vi "Configure Measurement.vi"(0 "VISA resource name":refnum<visa-resource-name>, 1 "Manual Resolution (2: 6.5 digits)":enum16{"4.5", "5.5", "6.5", "7.5", "8.5"}(ring)=enum."6.5", 5 "Function (0: DC Voltage)":u16(ring) items=["DC Voltage", "AC Voltage", "AC + DC Voltage", "DC Current", "AC Current", "AC + DC Current", "2-Wire Resistance", "4-Wire Resistance", "Frequency", "Period", "Direct Sampling DC", "Direct Sampling AC", "Sub-Sampling DC", "Sub-Sampling AC"], 7 "Frequency Source (3: AC Voltage)":u16(ring)=3 items=["AC + DC Current", "AC + DC Voltage", "AC Current", "AC Voltage"], 9 "Auto Range (1:ON)":u16(ring)=1 items=["OFF", "ON", "ONCE"], 11 "error in (no error)":errorcluster, 12 "Manual Range (1.00)":dbl=1.0 format="%_3g") -> (4 "VISA resource name out":refnum<visa-resource-name>, 15 "error out":errorcluster)   [LabVIEW 2020, in "3458A Basic Driver.lvlib"]
doc: "Configures the measurement type, resolution, range on the instrument and frequency source. Note that when setting for sub-sampling, you must specify a range, auto range cannot be used with sub-sampling. Also note that setting the integration cycle to a value greater than or equal to one prior to setting the manual resolution will result in the instrument setting the manual resolution to the highest number of digits for the function chosen regardless of user input. So if the user sets the number of integration cycles to one for DCV, the instrument will set the manual resolution to 8.5 digits even if the user sets it to 6.5 digits."
uses:
  3458A Basic Driver.lvlib
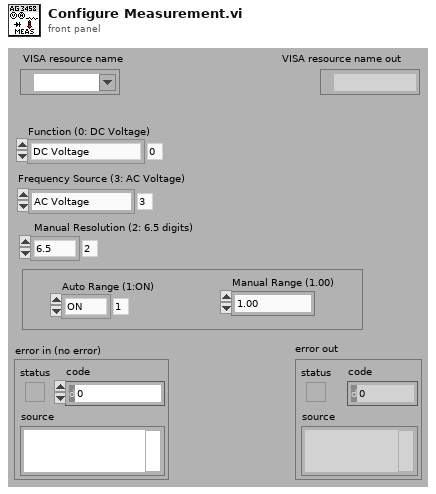
[diagram p1: front panel]
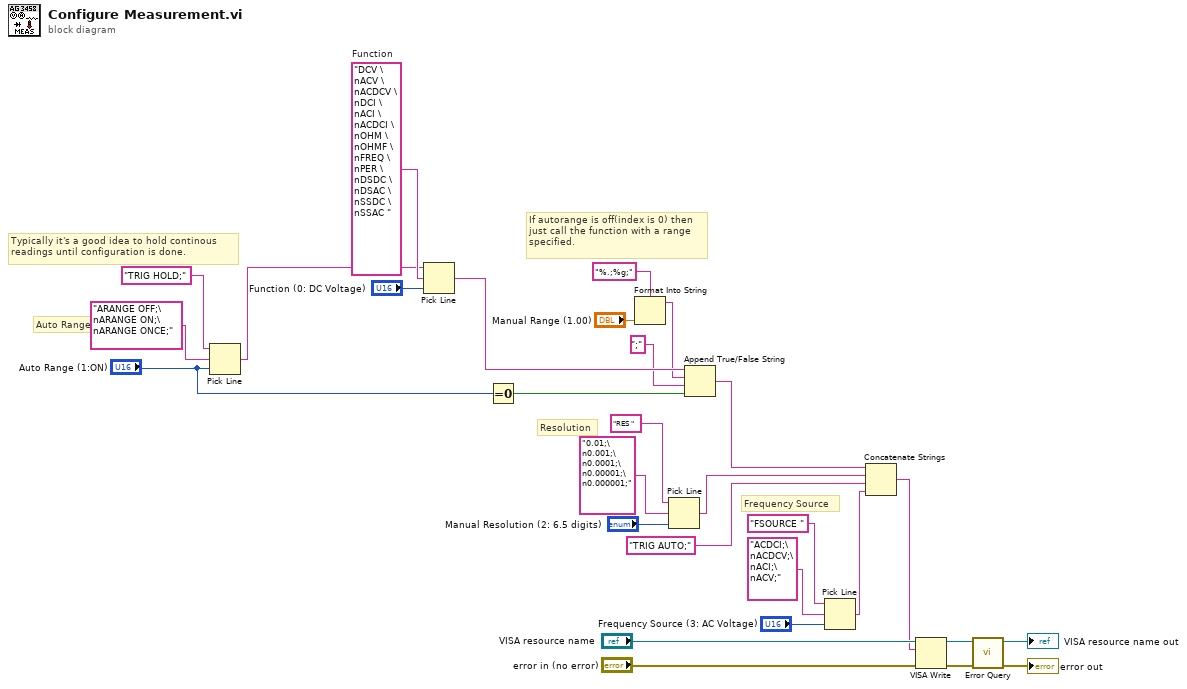
[diagram p0: block diagram]
diagram:
  w28 = "DCV \nACV \nACDCV \nDCI \nACI \nACDCI \nOHM \nOHMF \nFREQ \nPER \nDSDC \nDSAC \nSSDC \nSSAC "  # Function
  # "Resolution"
  # "Frequency Source"
  # "If autorange is off(index is 0) then\njust call the function with a range\nspecified."
  # "Typically it's a good idea to hold continous\nreadings until configuration is done."
  # "Auto Range"
  n1 = Pick Line(string ("")="TRIG HOLD;", multi-line string="ARANGE OFF;\nARANGE ON;\nARANGE ONCE;", line index="Auto Range (1:ON)") -> (output string=w23:string)
  n2 = Pick Line(string ("")=w23, multi-line string=w28, line index="Function (0: DC Voltage)") -> (output string=w14:string)
  n3 = Equal To 0?(x="Auto Range (1:ON)") -> (x = 0?=w13:bool)
  n4 = Format Into String(format string="%.;%g;", "Manual Range (1.00)") -> (resulting string=w12:string)  [unwired: 2 in, 1 out]
  n5 = Pick Line(string ("")="RES ", multi-line string="0.01;\n0.001;\n0.0001;\n0.00001;\n0.000001;", line index="Manual Resolution (2: 6.5 digits)") -> (output string=w6:string)
  n6 = Append True/False String(1:w13, 2:";", 3:w12, 4:w14) -> (0:w10:string)
  n7 = Pick Line(string ("")="FSOURCE ", multi-line string="ACDCI;\nACDCV;\nACI;\nACV;", line index="Frequency Source (3: AC Voltage)") -> (output string=w3:string)
  n8 = Concatenate Strings(w10, w6, "TRIG AUTO;", w3) -> (w2:string)
  n9 = VISA Write(VISA resource name="VISA resource name", write buffer=w2, error in (no error)="error in (no error)") -> (VISA resource name out=w18:refnum<visa-resource-name>, error out=w17:errorcluster)  [unwired: 1 out]
  n10 = call "Error Query.vi"("error in (no error)"=w17, "VISA resource name"=w18) -> ("error out"=→"error out":errorcluster, "VISA resource name out"=→"VISA resource name out":refnum<visa-resource-name>)  [unwired: 6 in, 2 out]
